vi "Subsys01_Global.vi"() -> ()   [LabVIEW 2019]
panel:
  out "S01_ST":u32(colorbox)
  out "S01_V01":dbl
  out "bos":bool
  out "spill_id":i64
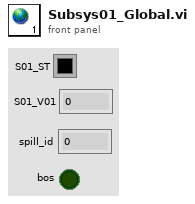
[diagram p1: front panel]
diagram:
